vi "ADIS16470 Accelerometer Angle Cal.vi"(10 "average samples":i32=1000, 11 "Raw Accel In":dbl[](array[numeric])) -> (1 "xAngle":dbl, 2 "yAngle":dbl, 3 "Average Accel Out":dbl[](array[numeric]))   [LabVIEW 2025]
uses:
  <vilib>/ptbypt/NI_PtbyPt.lvlib
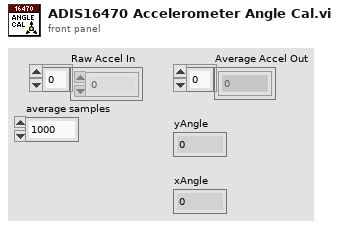
[diagram p1: front panel]
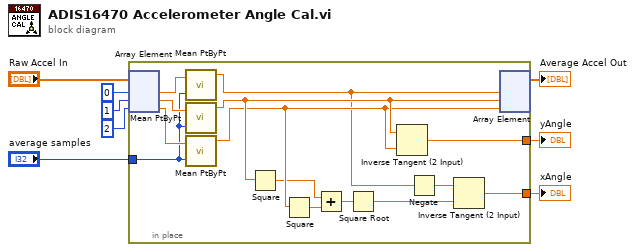
[diagram p0: block diagram]
diagram:
  n1 = in-place {
    in-place-border: [w19] -> w8
    in-place-border: [w10] -> w2
    in-place-border: "average samples" -> [w9]
    n2 = in-place-array #1("Raw Accel In", 0, 1, 2) -> (w22:dbl, w21:dbl, w20:dbl)
    n3 = call <vilib>:"Mean PtByPt.vi"("x"=w22, "sample length"=w9) -> ("mean"=w12:dbl)  [unwired: 2 in, 1 out]
    n4 = call <vilib>:"Mean PtByPt.vi"("x"=w21, "sample length"=w9) -> ("mean"=w18:dbl)  [unwired: 2 in, 1 out]
    n5 = call <vilib>:"Mean PtByPt.vi"("x"=w20, "sample length"=w9) -> ("mean"=w17:dbl)  [unwired: 2 in, 1 out]
    n6 = Square(x=w18) -> (x^2=w15:dbl)
    n7 = Square(x=w17) -> (x^2=w16:dbl)
    n8 = Add(x=w15, y=w16) -> (x+y=w14:dbl)
    n9 = Square Root(x=w14) -> (sqrt(x)=w13:dbl)
    n10 = Inverse Tangent (2 Input)(1:w17, 2:w18) -> (0:w19:dbl)
    n11 = Negate(x=w12) -> (-x=w11:dbl)
    n12 = Inverse Tangent (2 Input)(1:w13, 2:w11) -> (0:w10:dbl)
    n13 = in-place-array #1(w12, w18, w17) -> (→"Average Accel Out":dbl[])  [unwired: 3 out]
  }
  "xAngle" <- w2
  "yAngle" <- w8
